vi "Calibrate Noise Figure.vi"(8 "error in (no error)":errorcluster, 9 "Maximum Delay (30000ms)":i32=30000, 11 "VISA resource name":refnum<visa-resource-name>) -> (0 "error out":errorcluster, 3 "VISA resource name out":refnum<visa-resource-name>)   [LabVIEW 2014, in "Agilent ESA PSA Series.lvlib"]
doc: "Calibrates the Noise Figure personality using the ENR values entered to the Calibration ENR Table. If <B>Common Table</B> control is enabled, Measurement ENR Table is used instead of the Calibration ENR Table.\n\n<B>Note:</B> \n\nThis VI is only valid in Noise Figure personality. Use <B>Switch Personality</B> VI to switch to Noise Figure before calling this VI.\n\nIf the calibration doesn't happen and the execution finishes, try increasing the delay inside the <B>Switch Personality</B> vi."
uses:
  Agilent ESA PSA Series.lvlib
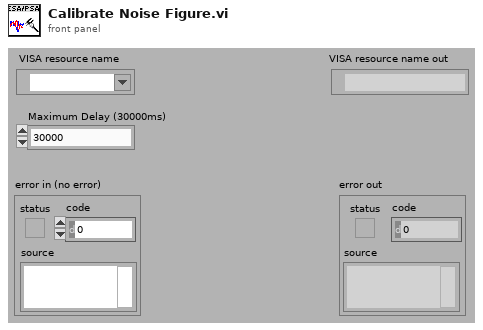
[diagram p1: front panel]
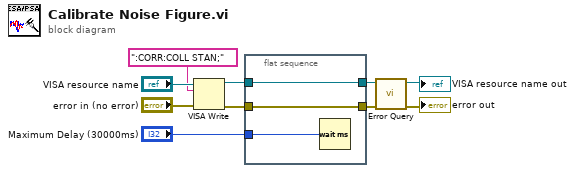
[diagram p0: block diagram]
diagram:
  n1 = VISA Write(VISA resource name="VISA resource name", write buffer=":CORR:COLL STAN;", error in (no error)="error in (no error)") -> (VISA resource name out=w5:refnum<visa-resource-name>, error out=w3:errorcluster)  [unwired: 1 out]
  n2 = flat-sequence {
    tunnel: [w13] -> w4
    tunnel: w5 -> [w13]
    tunnel: [w12] -> w2
    tunnel: w3 -> [w12]
    tunnel: "Maximum Delay (30000ms)" -> [w11]
    frame #0 {
      n3 = Wait (ms)(milliseconds to wait=w11) -> ()  [unwired: 1 out]
    }
  }
  n4 = call "Error Query.vi"("error in (no error)"=w2, "VISA resource name"=w4) -> ("error out"=→"error out":errorcluster, "VISA resource name out"=→"VISA resource name out":refnum<visa-resource-name>)  [unwired: 6 in, 2 out]
